vi "set initial state.vi"(10 "state module configuration.initial state":u8, 11 "tag bus configurable plugin module configuration in":refnum<class "user tag bus module configuration.lvclass">) -> (3 "tag bus configurable plugin module configuration out":refnum<class "user tag bus module configuration.lvclass">)   [LabVIEW 2013, in "user tag bus module configuration.lvclass"]
uses:
  user tag bus module configuration.lvclass
  user tag bus module configuration.lvclass/user tag bus module configuration.ctl
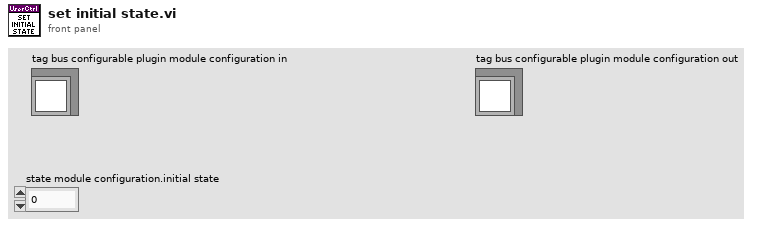
[diagram p1: front panel]
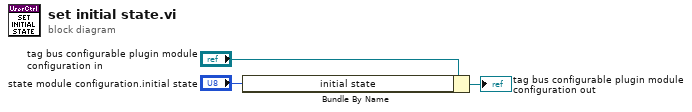
[diagram p0: block diagram]
diagram:
  n1 = Bundle By Name(cluster="tag bus configurable plugin module configuration in", "initial state"="state module configuration.initial state") -> (→"tag bus configurable plugin module configuration out":refnum<class "user tag bus module configuration.lvclass">)
